vi "TxtFile Save.vi"(8 "error in (no error)":errorcluster, 10 "text":string, 11 "Path":path) -> (0 "error out":errorcluster)   [LabVIEW 2012]
doc: "Use this template to build a VI to use as a subVI."
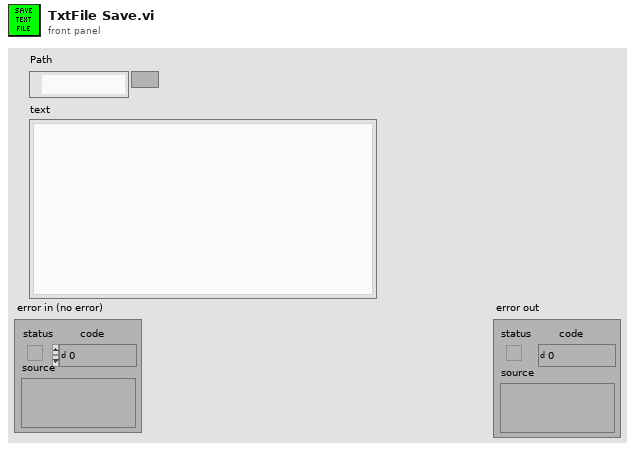
[diagram p1: front panel]
types:
  T1 = enum16{"open", "replace", "create", "open or create", "replace or create", "replace or create with confirmation"}
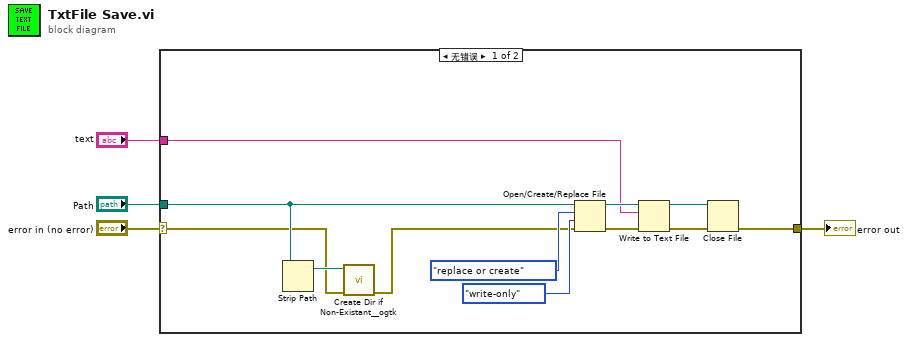
[diagram p0: block diagram]
diagram:
  n1 = case shown="无错误" "error in (no error)" {
    selector: "error in (no error)" -> [w6 w17]
    tunnel: [w10 w17] -> w3
    tunnel: "Path" -> [w8 _]
    tunnel: "text" -> [w9 _]
    frame No Error {
      n2 = Strip Path(path=w8) -> (stripped path=w7:path)  [unwired: 1 out]
      n3 = call <userlib>:"Create Dir if Non-Existant__ogtk.vi"("error in (no error)"=w6, "Directory Path"=w7) -> ("error out"=w5:errorcluster)  [unwired: 7 in, 2 out]
      n4 = Open/Create/Replace File(file path (use dialog)=w8, error in=w5, operation (0:open)=T1."replace or create", access (0:read/write)=enum16{"read/write", "read-only", "write-only"}."write-only") -> (refnum out=w14:refnum<file>, error out=w11:errorcluster)  [unwired: 2 in, 1 out]
      n5 = Write to Text File(file (use dialog)=w14, text=w9, error in=w11) -> (refnum out=w13:refnum<file>, error out=w12:errorcluster)  [unwired: 1 in, 1 out]
      n6 = Close File(refnum=w13, error in=w12) -> (error out=w10:errorcluster)  [unwired: 1 out]
    }
    frame Error {
    }
  }
  "error out" <- w3
